vi "周期设置_多参数.vi"() -> ()   [LabVIEW 2016, in "国弘多参数.lvlib"]
uses:
  <vilib>/Utility/miscctls.llb/LVPointTypeDef.ctl
  <vilib>/Utility/config.llb/NI_LVConfig.lvlib
panel:
  in  "运行周期":T1
  # "运行模式："
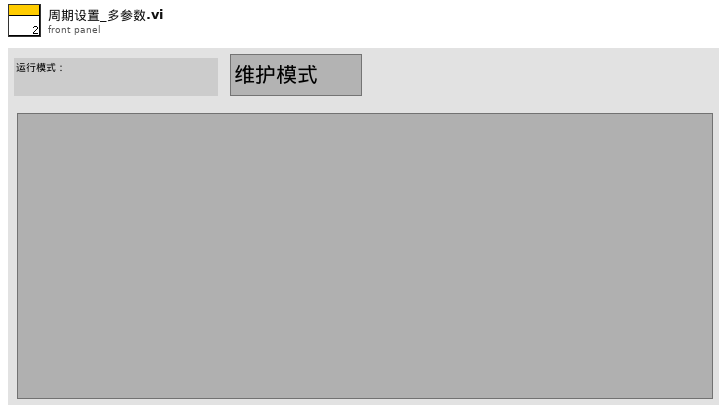
[diagram p1: front panel]
types:
  T1 = cluster{"运行模式":enum16{"维护模式", "常规模式", "应急模式", "质控模式"}, "24H周期设置":bool[]}
  T2 = typedef "LVPointTypeDef.ctl" = cluster{"Horizontal":i16, "Vertical":i16}
  T3 = enum16{"待机", "水样测试", "标样核查", "零点核查", "跨度核查", "空白测试", "平行样测试", "加标回收", "空白校准", "标样校准", "初始化（清洗）"}
  T4 = cluster{"测量模式":enum16{"待机", "水样测试", "标样核查", "零点核查", "跨度核查", "空白测试", "平行样测试", "加标回收", "空白校准", "标样校准", "初始化（清洗）"}, "数据标记表":string, "测量时间":dbl}
  T5 = typedef "LVDateTimeRec.ctl" = cluster{"秒数的小数部分":dbl, "秒":i32, "分":i32, "时":i32, "日":i32, "月":i32, "年":i32, "天数（周）":i32, "天数（年）":i32, "DST":i32}
  T6 = enum32{"Bad", "Idle", "Run top level", "Running"}
  T7 = typedef "NI_LVConfig.lvlib/Config Data RefNum.ctl" = refnum<k1>
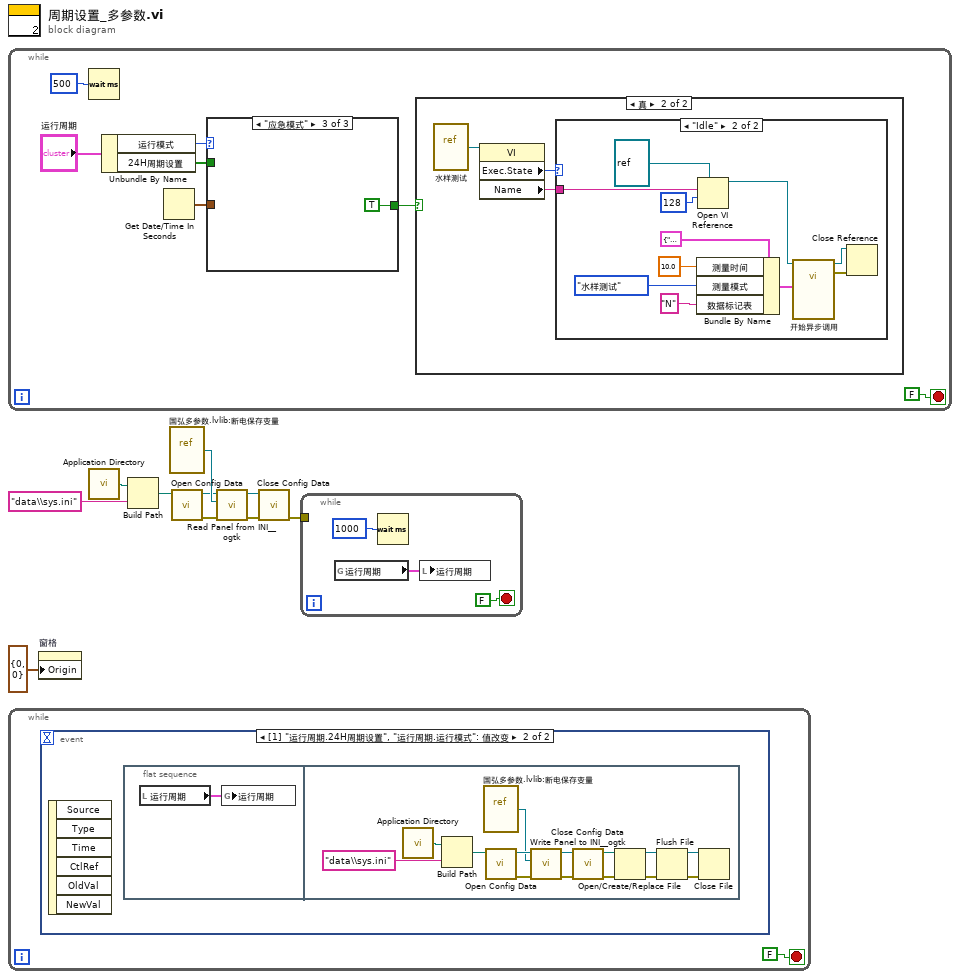
[diagram p0: block diagram]
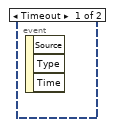
[diagram p2: hidden frame]
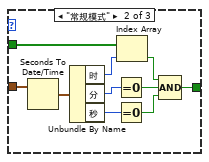
[diagram p6: hidden frame]
diagram:
  n1 = while {
    stop <- FALSE stop-if-true
    n2 = Wait (ms)(milliseconds to wait=u32 500 ("等待时间（毫秒）")) -> ()  [unwired: 1 out]
    n3 = Unbundle By Name("运行周期") -> ("运行模式"=w13:enum16{"维护模式", "常规模式", "应急模式", "质控模式"}, "24H周期设置"=w12:bool[])
    n4 = Get Date/Time In Seconds() -> (seconds since 1Jan1904=w17:timestamp)
    n5 = case shown="\"应急模式\"" w13 {
      tunnel: w17 -> [_ w41 _]
      tunnel: w12 -> [_ w38 _]
      tunnel: [_ w32 TRUE] -> w11
      frame "维护模式", Default {
      }
      frame "常规模式" {
        n6 = Seconds To Date/Time(time stamp (now)=w41) -> (date time rec=w40:T5)  [unwired: 1 in]
        n7 = Unbundle By Name(w40) -> ("时"=w39:i32, "分"=w37:i32, "秒"=w36:i32)
        n8 = Equal To 0?(x=w37) -> (x = 0?=w34:bool)
        n9 = Equal To 0?(x=w36) -> (x = 0?=w33:bool)
        n10 = Index Array(array=w38, index=w39) -> (element=w35:bool)
        n11 = Compound Arithmetic op=AND ("复合运算")(w35, w34, w33) -> (w32:bool)
      }
      frame "应急模式" {
      }
    }
    n12 = case shown="真" w11 {
      frame False {
      }
      frame True {
        n13 = vi-ref "水样测试.vi"() -> (w19:refnum<vi>)
        n14 = property class="VI"(reference=w19) -> ("Exec.State"=w18:T6, "Name"=w20:string)  [unwired: 1 in, 2 out]
        n15 = case shown="\"Idle\"" w18 {
          tunnel: w20 -> [_ w28]
          frame "Bad", Default {
          }
          frame "Idle" {
            n16 = Bundle By Name(cluster=T4 {"测量模式"=enum."待机", "数据标记表"="", "测量时间"=0.0} ("启动参数"), "测量时间"=10.0, "测量模式"=T3."水样测试", "数据标记表"="N") -> (w24:T4)
            n17 = Open VI Reference(type specifier VI Refnum (for type only)=refnum<vi> refnum, vi path=w28, options=128 ("选项")) -> (vi reference=w29:refnum<vi>)  [unwired: 3 in, 1 out]
            n18 = call-by-ref "开始异步调用"(reference=w29, "启动参数"=w24) -> (reference out=w30:refnum<vi>, error out=w31:errorcluster)  [unwired: 12 in]
            n19 = Close Reference(reference=w30, error in (no error)=w31) -> ()  [unwired: 1 out]
          }
        }
      }
    }
  }
  n20 = while {
    stop <- FALSE stop-if-true
    n21 = event shown="[1] \"运行周期.24H周期设置\", \"运行周期.运行模式\": 值改变" {
      selector: _ -> [_ _]
      dyn-events: _ -> [_ _]
      timeout: _ -> [_ _]
      event Timeout {
        n22 = event-data() -> ()  [unwired: 1 in, 3 out]
      }
      event "运行周期.24H周期设置", "运行周期.运行模式": Value Change {
        n23 = event-data() -> ()  [unwired: 1 in, 6 out]
        n24 = flat-sequence {
          frame #0 {
            n25 = local read "运行周期"() -> (w44:T1)
            n26 = global write "断电保存变量.vi" "运行周期"(w44) -> ()
          }
          frame #1 {
            n27 = call <vilib>:"Application Directory.vi"() -> ("Application Directory"=w58:path)
            n28 = Build Path(base path=w58, name or relative path="data\\sys.ini" ("名称或相对路径")) -> (appended path=w56:path)
            n29 = vi-ref "国弘多参数.lvlib:断电保存变量.vi"() -> (w54:refnum<vi>)
            n30 = call <vilib>:"Open Config Data.vi"("configuration file path"=w56) -> ("error out"=w52:errorcluster, "refnum"=w55:T7)  [unwired: 8 in, 1 out]
            n31 = call <userlib>:"Write Panel to INI__ogtk.vi"("error in (no error)"=w52, "VI ref"=w54, "refnum"=w55) -> ("error out"=w51:errorcluster, "refnum out"=w53:T7)  [unwired: 7 in]
            n32 = call <vilib>:"Close Config Data.vi"("error in (no error)"=w51, "refnum"=w53) -> ("error out"=w46:errorcluster, "file path"=w45:path)  [unwired: 8 in]
            n33 = Open/Create/Replace File(file path (use dialog)=w45, error in=w46) -> (refnum out=w49:refnum<file>, error out=w50:errorcluster)  [unwired: 4 in, 1 out]
            n34 = Flush File(refnum=w49, error in=w50) -> (refnum out=w48:refnum<file>, error out=w47:errorcluster)
            n35 = Close File(refnum=w48, error in=w47) -> ()  [unwired: 2 out]
          }
        }
      }
    }
  }
  n36 = property on="窗格" class="Pane"("Origin"=T2 {"Horizontal"=0, "Vertical"=0} ("原点")) -> ()  [unwired: 2 in, 2 out]
  n37 = call <vilib>:"Application Directory.vi"() -> ("Application Directory"=w3:path)
  n38 = Build Path(base path=w3, name or relative path="data\\sys.ini" ("名称或相对路径")) -> (appended path=w5:path)
  n39 = vi-ref "国弘多参数.lvlib:断电保存变量.vi"() -> (w7:refnum<vi>)
  n40 = call <vilib>:"Open Config Data.vi"("configuration file path"=w5) -> ("error out"=w9:errorcluster, "refnum"=w6:T7)  [unwired: 8 in, 1 out]
  n41 = call <userlib>:"Read Panel from INI__ogtk.vi"("error in (no error)"=w9, "VI ref"=w7, "refnum"=w6) -> ("error out"=w10:errorcluster, "refnum out"=w8:T7)  [unwired: 7 in]
  n42 = call <vilib>:"Close Config Data.vi"("error in (no error)"=w10, "refnum"=w8) -> ("error out"=w2:errorcluster)  [unwired: 8 in, 1 out]
  n43 = while {
    tunnel: w2 -> [_]
    stop <- FALSE stop-if-true
    n44 = global read "断电保存变量.vi" "运行周期"() -> (w59:T1)
    n45 = Wait (ms)(milliseconds to wait=u32 1000 ("等待时间（毫秒）")) -> ()  [unwired: 1 out]
    n46 = local write "运行周期"(w59) -> ()
  }
